vi "write_results.vi"(8 "error in (no error)":errorcluster, 10 "Labelled Integrals":T1(array[cluster]), 11 "file path":path) -> (0 "error out":errorcluster)   [LabVIEW 2020]
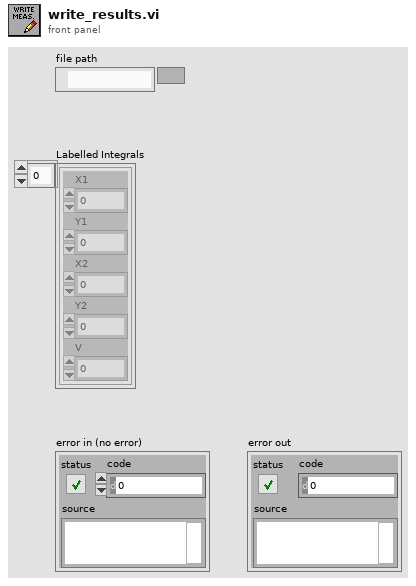
[diagram p1: front panel]
types:
  T1 = cluster{"X1":dbl, "Y1":dbl, "X2":dbl, "Y2":dbl, "V":dbl}[]
  T2 = enum16{"open", "replace", "create", "open or create", "replace or create", "replace or create with confirmation"}
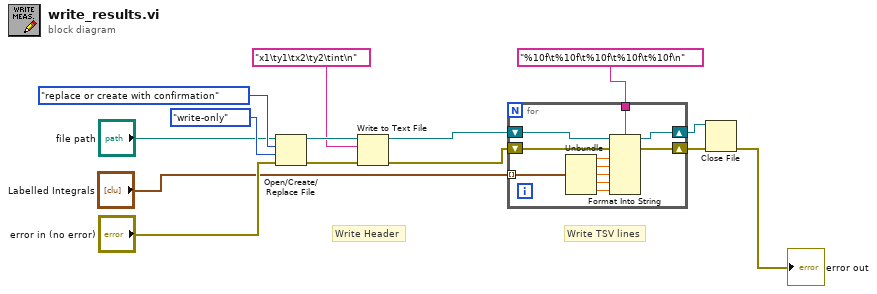
[diagram p0: block diagram]
diagram:
  # "Write TSV lines"
  # "Write Header"
  n1 = Open/Create/Replace File(file path (use dialog)="file path", error in="error in (no error)", operation (0:open)=T2."replace or create with confirmation", access (0:read/write)=enum16{"read/write", "read-only", "write-only"}."write-only") -> (refnum out=w5:refnum<file>, error out=w2:errorcluster)  [unwired: 2 in, 1 out]
  n2 = Write to Text File(file (use dialog)=w5, text="x1\ty1\tx2\ty2\tint\n", error in=w2) -> (refnum out=w4:refnum<file>, error out=w3:errorcluster)  [unwired: 1 in, 1 out]
  n3 = for {
    tunnel: "Labelled Integrals" -> [w25] mode=indexing
    shift-right: [w17] -> w13
    shift-left: w3 -> [w18]
    shift-right: [w16] -> w12
    shift-left: w4 -> [w19]
    tunnel: "%10f\t%10f\t%10f\t%10f\t%10f\n" ("format string") -> [w15]
    n4 = Unbundle(w25) -> ("X1"=w24:dbl, "Y1"=w23:dbl, "X2"=w22:dbl, "Y2"=w21:dbl, "V"=w20:dbl)
    n5 = Format Into String(format string=w15, initial string=w19, error in=w18, w24, w23, w22, w21, w20) -> (resulting string=w16:refnum<file>, error out=w17:errorcluster)
  }
  n6 = Close File(refnum=w12, error in=w13) -> (error out=→"error out":errorcluster)  [unwired: 1 out]
